vi "1A2B.vi"() -> ()   [LabVIEW 2019]
panel:
  out "Guess Times":i16
  out "Boolean":bool
  out "result 2":bool
  in  "Numeric Control 4":i8 min=0 max=9
  in  "Numeric Control 3":i8 min=0 max=9
  in  "Numeric Control 2":i8 min=0 max=9
  in  "Numeric Control":i8 min=0 max=9
  in  ".NET Container":refnum<k24>(container)
  out "猜過的數字列表":string[][](array[string])
  out "Time now 2":i16
  out "Time now":i16
  in  "stop 2":bool
  in  "Guess":bool
  out "Answer":i16[](array[numeric]) min=0 max=9
  in  ".NET Container 2":refnum<k24>(container)
  # "分"
  # "秒"
  # "Guess Times ："
  # "Time："
  # "Guess Number："
  # "Correct Answer："
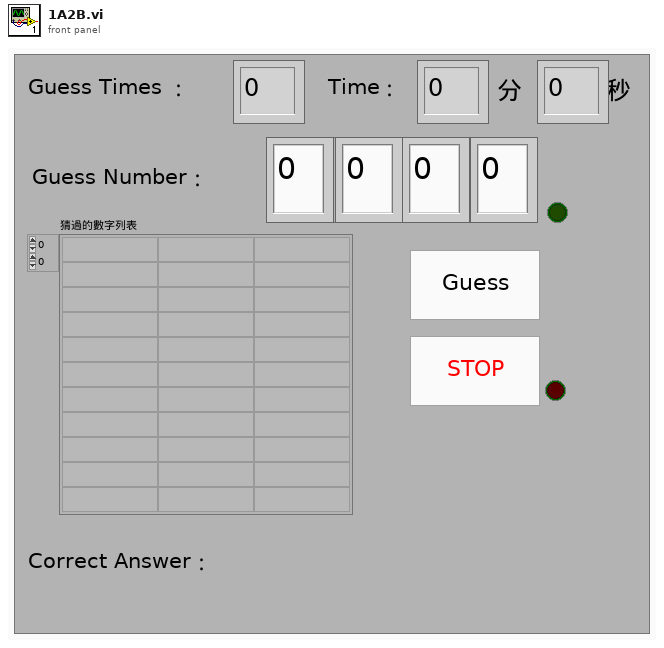
[diagram p1: front panel]
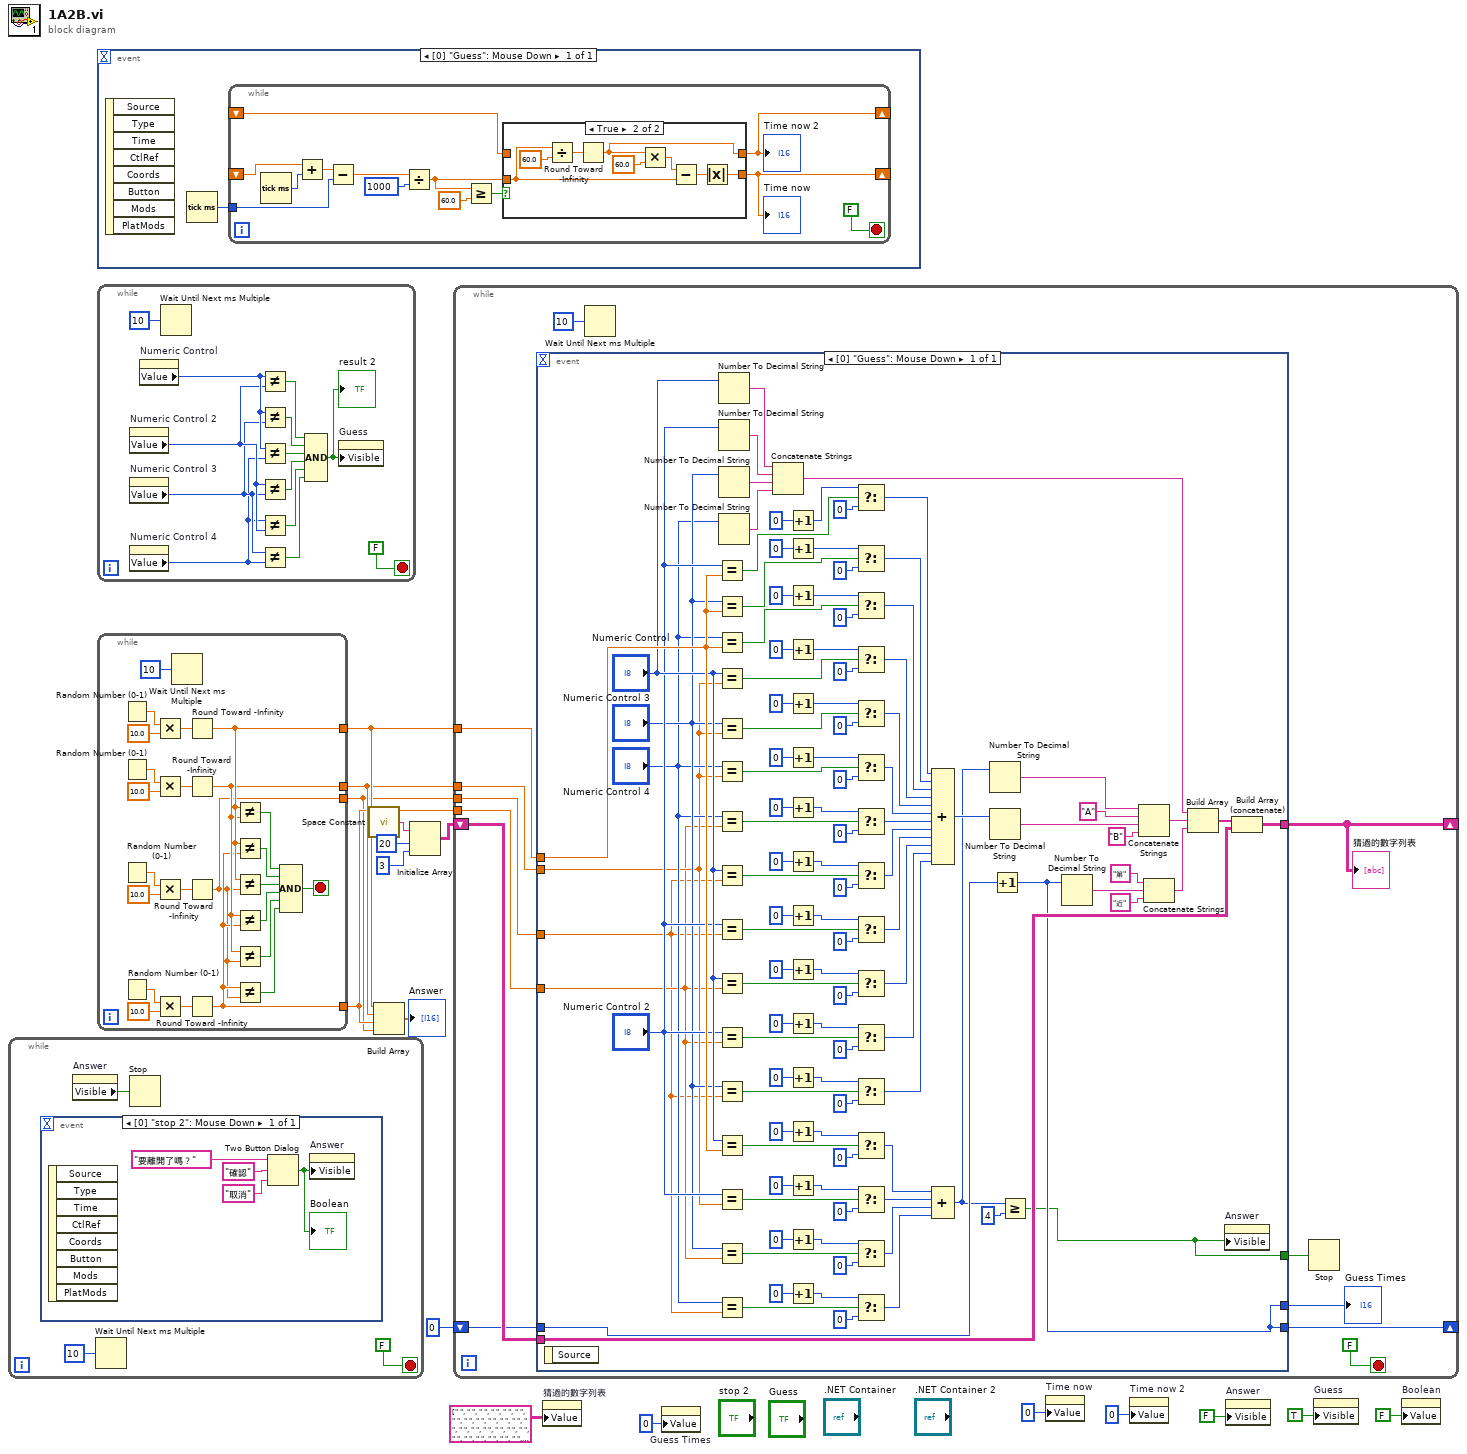
[diagram p0: block diagram]
diagram:
  n1 = while {
    stop <- FALSE stop-if-true
    n2 = event shown="[0] \"stop 2\": Mouse Down" {
      selector: _ -> [_]
      dyn-events: _ -> [_]
      timeout: _ -> [_]
      event "stop 2": Mouse Down {
        n3 = event-data() -> ()  [unwired: 1 in, 8 out]
        n4 = Two Button Dialog(message="要離開了嗎？", 1:"取消" ("F button name (\"Cancel\")"), 2:"確認" ("T button name (\"OK\")")) -> (T button?=w21:bool)
        "Boolean" <- w21
        n5 = property on="Answer" class="Arr (strict)"("Visible"=w21) -> ()  [unwired: 2 in, 2 out]
      }
    }
    n6 = property on="Answer" class="Arr (strict)"() -> ("Visible"=w20:bool)  [unwired: 2 in, 2 out]
    n7 = Wait Until Next ms Multiple(millisecond multiple=u32 10) -> ()  [unwired: 1 out]
    n8 = Stop(stop? (T)=w20) -> ()
  }
  n9 = event shown="[0] \"Guess\": Mouse Down" {
    selector: _ -> [_]
    dyn-events: _ -> [_]
    timeout: _ -> [_]
    event "Guess": Mouse Down {
      n10 = event-data() -> ()  [unwired: 1 in, 8 out]
      n11 = Tick Count (ms)() -> (millisecond timer value=w25:u32)
      n12 = while {
        tunnel: w25 -> [w38]
        shift-right: [w30] -> _
        shift-left: _ -> [w34]
        shift-right: [w28] -> _
        shift-left: _ -> [w29]
        stop <- FALSE stop-if-true
        n13 = Tick Count (ms)() -> (millisecond timer value=w27:u32)
        n14 = Add(x=w34, y=w27) -> (x+y=w35:dbl)
        n15 = Subtract(x=w35, y=w38) -> (x-y=w37:dbl)
        n16 = Divide(x=w37, y=u32 1000) -> (x/y=w31:dbl)
        n17 = Greater Or Equal?(x=w31, y=60.0) -> (x >= y?=w32:bool)
        n18 = case shown="True" w32 {
          tunnel: [w40 w41] -> w30
          tunnel: w31 -> [w40 w45]
          tunnel: w29 -> [w39 _]
          tunnel: [w39 w43] -> w28
          frame False {
          }
          frame True {
            n19 = Divide(x=w45, y=60.0) -> (x/y=w44:dbl)
            n20 = Round Toward -Infinity(1:w44) -> (0:w43:dbl)
            n21 = Multiply(x=w43, y=60.0) -> (x*y=w46:dbl)
            n22 = Subtract(x=w46, y=w45) -> (x-y=w42:dbl)
            n23 = Absolute Value(x=w42) -> (abs(x)=w41:dbl)
          }
        }
        "Time now" <- w30
        "Time now 2" <- w28
      }
    }
  }
  n24 = while {
    stop <- FALSE stop-if-true
    n25 = property on="Numeric Control 2" class="DigNum (strict)"() -> ("Value"=w60:i8)  [unwired: 2 in, 2 out]
    n26 = property on="Numeric Control 3" class="DigNum (strict)"() -> ("Value"=w59:i8)  [unwired: 2 in, 2 out]
    n27 = property on="Numeric Control 4" class="DigNum (strict)"() -> ("Value"=w58:i8)  [unwired: 2 in, 2 out]
    n28 = property on="Numeric Control" class="DigNum (strict)"() -> ("Value"=w61:i8)  [unwired: 2 in, 2 out]
    n29 = Wait Until Next ms Multiple(millisecond multiple=u32 10) -> ()  [unwired: 1 out]
    n30 = Not Equal?(x=w61, y=w60) -> (x != y?=w50:bool)
    n31 = Not Equal?(x=w61, y=w59) -> (x != y?=w51:bool)
    n32 = Not Equal?(x=w61, y=w58) -> (x != y?=w52:bool)
    n33 = Not Equal?(x=w60, y=w59) -> (x != y?=w53:bool)
    n34 = Not Equal?(x=w58, y=w60) -> (x != y?=w54:bool)
    n35 = Not Equal?(x=w59, y=w58) -> (x != y?=w55:bool)
    n36 = Compound Arithmetic op=AND(w50, w51, w52, w53, w54, w55) -> (w56:bool)
    "result 2" <- w56
    n37 = property on="Guess" class="Bool (strict)"("Visible"=w56) -> ()  [unwired: 2 in, 2 out]
  }
  n38 = while {
    tunnel: [w66] -> w11
    tunnel: [w65] -> w10
    tunnel: [w64] -> w9
    tunnel: [w62] -> w8
    stop <- w67 stop-if-true
    n39 = Random Number (0-1)() -> (number: 0 to 1=w85:dbl)
    n40 = Random Number (0-1)() -> (number: 0 to 1=w83:dbl)
    n41 = Random Number (0-1)() -> (number: 0 to 1=w77:dbl)
    n42 = Random Number (0-1)() -> (number: 0 to 1=w79:dbl)
    n43 = Multiply(x=w85, y=10.0) -> (x*y=w84:dbl)
    n44 = Multiply(x=w83, y=10.0) -> (x*y=w82:dbl)
    n45 = Multiply(x=w77, y=10.0) -> (x*y=w76:dbl)
    n46 = Multiply(x=w79, y=10.0) -> (x*y=w78:dbl)
    n47 = Wait Until Next ms Multiple(millisecond multiple=u32 10) -> ()  [unwired: 1 out]
    n48 = Round Toward -Infinity(1:w84) -> (0:w66:dbl)
    n49 = Round Toward -Infinity(1:w82) -> (0:w65:dbl)
    n50 = Round Toward -Infinity(1:w76) -> (0:w62:dbl)
    n51 = Round Toward -Infinity(1:w78) -> (0:w64:dbl)
    n52 = Not Equal?(x=w66, y=w65) -> (x != y?=w73:bool)
    n53 = Not Equal?(x=w66, y=w64) -> (x != y?=w72:bool)
    n54 = Not Equal?(x=w66, y=w62) -> (x != y?=w71:bool)
    n55 = Not Equal?(x=w65, y=w64) -> (x != y?=w70:bool)
    n56 = Not Equal?(x=w65, y=w62) -> (x != y?=w69:bool)
    n57 = Not Equal?(x=w64, y=w62) -> (x != y?=w68:bool)
    n58 = Compound Arithmetic op=AND(w73, w72, w71, w70, w69, w68) -> (w67:bool)
  }
  n59 = call <vilib>:"Space Constant.vi"() -> ("String"=w14:string)
  n60 = Build Array(w11, w10, w9, w8) -> (→"Answer":dbl[])
  n61 = Initialize Array(w14, 20 ("dimension size"), 3 ("dimension size")) -> (w15:string[][])
  n62 = while {
    shift-right: [w89] -> _
    shift-left: w15 -> [w97]
    shift-right: [w95] -> _
    shift-left: 0 -> [w96]
    tunnel: w11 -> [w94]
    tunnel: w10 -> [w93]
    tunnel: w9 -> [w92]
    tunnel: w8 -> [w91]
    stop <- FALSE stop-if-true
    n63 = event shown="[0] \"Guess\": Mouse Down" {
      selector: _ -> [_]
      dyn-events: _ -> [_]
      timeout: _ -> [_]
      tunnel: [w198] -> w89
      tunnel: w97 -> [w197]
      tunnel: w96 -> [w192]
      tunnel: [w99] -> w95
      tunnel: [w99] -> w86
      tunnel: w94 -> [w195]
      tunnel: w93 -> [w186]
      tunnel: w92 -> [w185]
      tunnel: w91 -> [w184]
      tunnel: [w98] -> w87
      event "Guess": Mouse Down {
        n64 = event-data() -> ()  [unwired: 1 in, 1 out]
        n65 = Equal?(x="Numeric Control 2", y=w195) -> (x = y?=w117:bool)
        n66 = Equal?(x="Numeric Control 3", y=w195) -> (x = y?=w116:bool)
        n67 = Equal?(x="Numeric Control 4", y=w195) -> (x = y?=w115:bool)
        n68 = Equal?(x="Numeric Control", y=w186) -> (x = y?=w114:bool)
        n69 = Equal?(x="Numeric Control 3", y=w186) -> (x = y?=w112:bool)
        n70 = Equal?(x="Numeric Control 4", y=w186) -> (x = y?=w111:bool)
        n71 = Equal?(x="Numeric Control 4", y=w185) -> (x = y?=w107:bool)
        n72 = Equal?(x="Numeric Control", y=w184) -> (x = y?=w106:bool)
        n73 = Equal?(x="Numeric Control 2", y=w184) -> (x = y?=w105:bool)
        n74 = Equal?(x="Numeric Control", y=w185) -> (x = y?=w110:bool)
        n75 = Equal?(x="Numeric Control 2", y=w185) -> (x = y?=w109:bool)
        n76 = Equal?(x="Numeric Control 3", y=w184) -> (x = y?=w104:bool)
        n77 = Equal?(x="Numeric Control", y=w195) -> (x = y?=w118:bool)
        n78 = Equal?(x="Numeric Control 2", y=w186) -> (x = y?=w113:bool)
        n79 = Equal?(x="Numeric Control 3", y=w185) -> (x = y?=w108:bool)
        n80 = Equal?(x="Numeric Control 4", y=w184) -> (x = y?=w103:bool)
        n81 = Number To Decimal String(number="Numeric Control") -> (decimal integer string=w203:string)  [unwired: 1 in]
        n82 = Number To Decimal String(number="Numeric Control 2") -> (decimal integer string=w204:string)  [unwired: 1 in]
        n83 = Number To Decimal String(number="Numeric Control 3") -> (decimal integer string=w205:string)  [unwired: 1 in]
        n84 = Number To Decimal String(number="Numeric Control 4") -> (decimal integer string=w206:string)  [unwired: 1 in]
        n85 = Concatenate Strings(w203, w204, w205, w206) -> (w207:string)
        n86 = Increment(x=0) -> (x+1=w176:i32)
        n87 = Increment(x=0) -> (x+1=w174:i32)
        n88 = Increment(x=0) -> (x+1=w172:i32)
        n89 = Increment(x=0) -> (x+1=w170:i32)
        n90 = Increment(x=0) -> (x+1=w162:i32)
        n91 = Increment(x=0) -> (x+1=w160:i32)
        n92 = Increment(x=0) -> (x+1=w148:i32)
        n93 = Increment(x=0) -> (x+1=w146:i32)
        n94 = Increment(x=0) -> (x+1=w140:i32)
        n95 = Increment(x=0) -> (x+1=w158:i32)
        n96 = Increment(x=0) -> (x+1=w152:i32)
        n97 = Increment(x=0) -> (x+1=w138:i32)
        n98 = Increment(x=0) -> (x+1=w182:i32)
        n99 = Increment(x=0) -> (x+1=w164:i32)
        n100 = Increment(x=0) -> (x+1=w150:i32)
        n101 = Increment(x=0) -> (x+1=w136:i32)
        n102 = Select(t=w176, s=w117, f=0) -> (s? t:f=w130:i32)
        n103 = Select(t=w174, s=w116, f=0) -> (s? t:f=w129:i32)
        n104 = Select(t=w172, s=w115, f=0) -> (s? t:f=w128:i32)
        n105 = Select(t=w170, s=w114, f=0) -> (s? t:f=w127:i32)
        n106 = Select(t=w162, s=w112, f=0) -> (s? t:f=w126:i32)
        n107 = Select(t=w160, s=w111, f=0) -> (s? t:f=w125:i32)
        n108 = Select(t=w148, s=w107, f=0) -> (s? t:f=w124:i32)
        n109 = Select(t=w146, s=w106, f=0) -> (s? t:f=w123:i32)
        n110 = Select(t=w140, s=w105, f=0) -> (s? t:f=w122:i32)
        n111 = Select(t=w158, s=w110, f=0) -> (s? t:f=w121:i32)
        n112 = Select(t=w152, s=w109, f=0) -> (s? t:f=w120:i32)
        n113 = Select(t=w138, s=w104, f=0) -> (s? t:f=w119:i32)
        n114 = Select(t=w182, s=w118, f=0) -> (s? t:f=w135:i32)
        n115 = Select(t=w164, s=w113, f=0) -> (s? t:f=w134:i32)
        n116 = Select(t=w150, s=w108, f=0) -> (s? t:f=w132:i32)
        n117 = Select(t=w136, s=w103, f=0) -> (s? t:f=w133:i32)
        n118 = Compound Arithmetic op=ADD(w130, w129, w128, w127, w126, w125, w124, w123, w122, w121, w120, w119) -> (w131:i32)
        n119 = Compound Arithmetic op=ADD(w135, w134, w132, w133) -> (w101:i32)
        n120 = Number To Decimal String(number=w101) -> (decimal integer string=w194:string)  [unwired: 1 in]
        n121 = Number To Decimal String(number=w131) -> (decimal integer string=w193:string)  [unwired: 1 in]
        n122 = Increment(x=w192) -> (x+1=w99:i32)
        n123 = Greater Or Equal?(x=w101, y=4) -> (x >= y?=w98:bool)
        n124 = Number To Decimal String(number=w99) -> (decimal integer string=w196:string)  [unwired: 1 in]
        n125 = Concatenate Strings(w194, "A" ("string"), w193, "B" ("string")) -> (w191:string)
        n126 = Concatenate Strings("第" ("string"), w196, "近" ("string")) -> (w208:string)
        n127 = Build Array(w207, w191, w208) -> (w102:string[])
        n128 = property on="Answer" class="Arr (strict)"("Visible"=w98) -> ()  [unwired: 2 in, 2 out]
        n129 = Build Array (concatenate)(w102, w197) -> (w198:string[][])
      }
    }
    "猜過的數字列表" <- w89
    "Guess Times" <- w86
    n130 = Wait Until Next ms Multiple(millisecond multiple=u32 10) -> ()  [unwired: 1 out]
    n131 = Stop(stop? (T)=w87) -> ()
  }
  n132 = property on="猜過的數字列表" class="Arr (strict)"("Value"=string[][] [[" ", " ", " "], [" ", " ", " "], [" ", " ", " "], [" ", " ", " "], [" ", " ", " "], [" ", " ", " "], [" ", " ", " "], [" ", " ", " "], [" ", " ", " "], [" ", " ", " "], [" ", " ", " "], [" ", " ", " "], [" ", " ", " "], [" ", " ", " "], [" ", " ", " "], [" ", " ", " "], [" ", " ", " "], [" ", " ", " "], [" ", " ", " "], [" ", " ", " "], [" ", " ", " "]] ("猜過的數字列表")) -> ()  [unwired: 2 in, 2 out]
  n133 = property on="Guess Times" class="DigNum (strict)"("Value"=i16 0 ("Guess Times")) -> ()  [unwired: 2 in, 2 out]
  n134 = property on="Time now" class="DigNum (strict)"("Value"=i16 0 ("Time now")) -> ()  [unwired: 2 in, 2 out]
  n135 = property on="Time now 2" class="DigNum (strict)"("Value"=i16 0 ("Time now 2")) -> ()  [unwired: 2 in, 2 out]
  n136 = property on="Answer" class="Arr (strict)"("Visible"=FALSE) -> ()  [unwired: 2 in, 2 out]
  n137 = property on="Guess" class="Bool (strict)"("Visible"=TRUE) -> ()  [unwired: 2 in, 2 out]
  n138 = property on="Boolean" class="Bool (strict)"("Value"=FALSE ("Boolean")) -> ()  [unwired: 2 in, 2 out]
